vi "TestParseSolverString.vi"() -> ()   [LabVIEW 2017]
panel:
  out "Array":u16[](array[numeric])
  in  "String":string
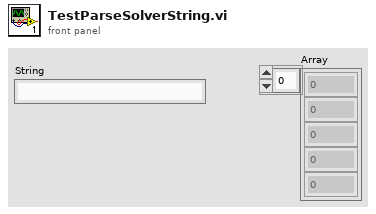
[diagram p1: front panel]
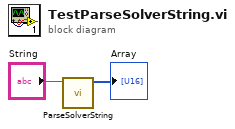
[diagram p0: block diagram]
diagram:
  n1 = call "ParseSolverString.vi"("String"="String") -> ("Array"=→"Array":u16[])  [unwired: 10 in]
